vi "Stanford Research CG635 Time Capture.vi"() -> ()   [LabVIEW 2013]
uses:
  <instrlib>/Stanford Research CG635/Stanford Research CG635.lvlib
panel:
  in  "Unit (MHz)":u16(ring)=1 items=["GHz", "MHz", "KHz", "Hz"]
  in  "Stop State (0)":u16(ring) items=["0", "1", "2"]
  in  "Running State (1)":u16(ring)=1 items=["0", "1"]
  in  "CMOS High (5 V)":dbl=5.0
  in  "CMOS Low (0 V)":dbl
  in  "?":bool
  in  "Phase (0°)":i32
  out "Waveform Chart":dbl(graph)=-1.0
  in  "Frequency (10.000000 MHz)":dbl=10.0
  in  "VISA resource name":refnum<visa-resource-name>
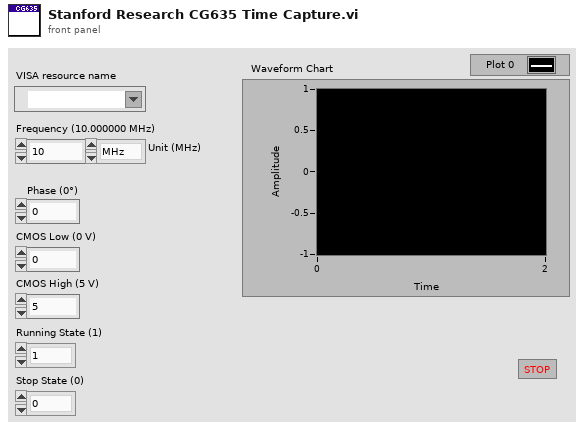
[diagram p1: front panel]
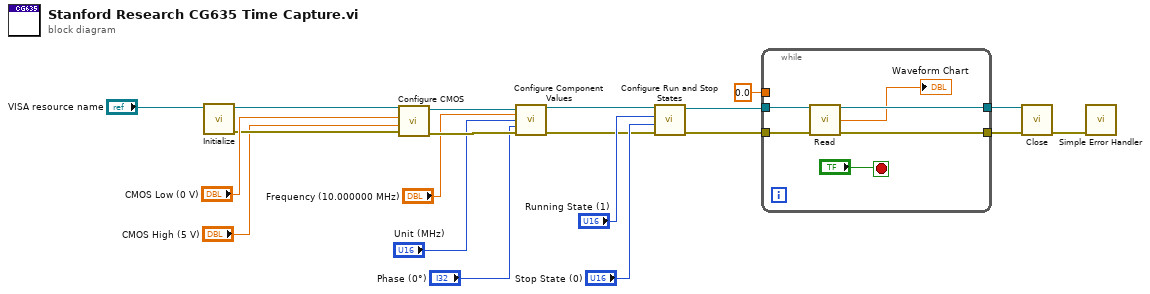
[diagram p0: block diagram]
diagram:
  n1 = call <instrlib>:"Initialize.vi"("VISA resource name"="VISA resource name") -> ("error out"=w13:errorcluster, "VISA resource name out"=w14:refnum<visa-resource-name>)  [unwired: 9 in]
  n2 = call <instrlib>:"Configure CMOS.vi"("error in (no error)"=w13, "CMOS High (5 V)"="CMOS High (5 V)", "CMOS Low (0 V)"="CMOS Low (0 V)", "VISA resource name"=w14) -> ("error out"=w6:errorcluster, "VISA resource name out"=w8:refnum<visa-resource-name>)  [unwired: 6 in]
  n3 = call <instrlib>:"Configure Component Values.vi"("VISA resource name"=w8, "Frequency (10.000000 MHz)"="Frequency (10.000000 MHz)", "Unit (MHz)"="Unit (MHz)", "Phase (0°)"="Phase (0°)", "error in (no error)"=w6) -> ("VISA resource name out"=w7:refnum<visa-resource-name>, "error out"=w5:errorcluster)  [unwired: 9 in]
  n4 = call <instrlib>:"Configure Run and Stop States.vi"("error in (no error)"=w5, "Stop State (0)"="Stop State (0)", "Running State (1)"="Running State (1)", "VISA resource name"=w7) -> ("error out"=w11:errorcluster, "VISA resource name out"=w12:refnum<visa-resource-name>)  [unwired: 6 in]
  n5 = while {
    tunnel: w11 -> [w25]
    tunnel: [w23] -> w18
    tunnel: 0.0 ("double precision float") -> [_]
    tunnel: w12 -> [w26]
    tunnel: [w24] -> w19
    stop <- "?" stop-if-true
    n6 = call <instrlib>:"Read.vi"("VISA resource name"=w26, "error in (no error)"=w25) -> ("VISA resource name out"=w24:refnum<visa-resource-name>, "double precision float"=→"Waveform Chart":dbl, "error out"=w23:errorcluster)  [unwired: 11 in]
  }
  n7 = call <instrlib>:"Close.vi"("error in (no error)"=w18, "VISA resource name"=w19) -> ("error out"=w17:errorcluster)  [unwired: 9 in]
  n8 = call <vilib>:"Simple Error Handler.vi"("error in (no error)"=w17) -> ()  [unwired: 4 in, 5 out]
